vi "UI Initialize.vi"(8 "error in (no error)":errorcluster, 11 "UI View in":refnum<class "UI View.lvclass">) -> (0 "error out":errorcluster, 3 "UI View out":refnum<class "UI View.lvclass">)   [LabVIEW 2013, in "SET Project Editor.lvlib" / "UI View.lvclass"]
uses:
  UI View.lvclass
panel:
  # "Call UI Initialize just before Actor Core.vi"
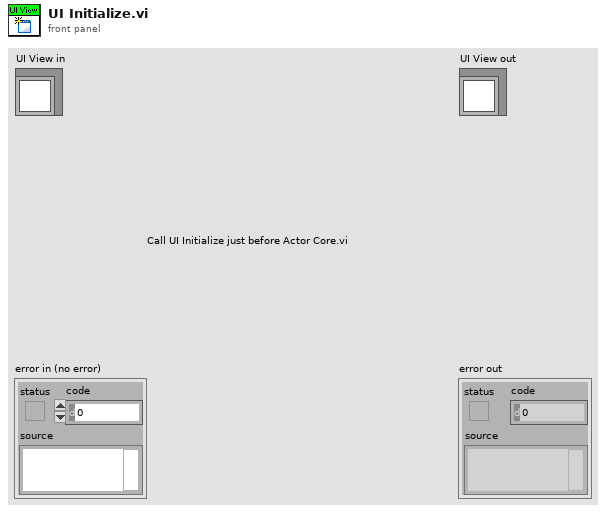
[diagram p1: front panel]
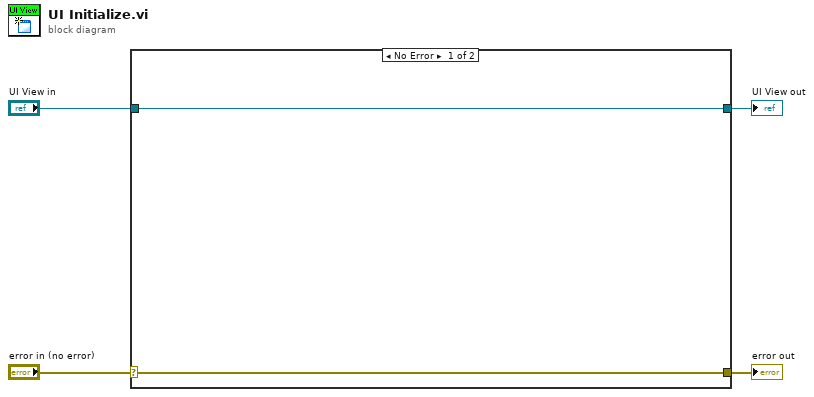
[diagram p0: block diagram]
diagram:
  n1 = case shown="No Error" "error in (no error)" {
    selector: "error in (no error)" -> [w5 w8]
    tunnel: [w5 w8] -> w3
    tunnel: [w6 w7] -> w1
    tunnel: "UI View in" -> [w6 w7]
    frame No Error {
    }
    frame Error {
    }
  }
  "error out" <- w3
  "UI View out" <- w1
